vi "G.vi"(9 "5":string[](array[string]), 10 "4":string, 11 "A":string) -> (3 "G":string)   [LabVIEW 2017]
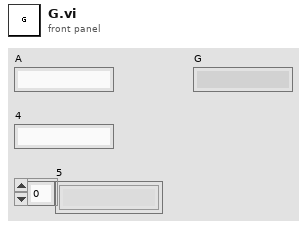
[diagram p1: front panel]
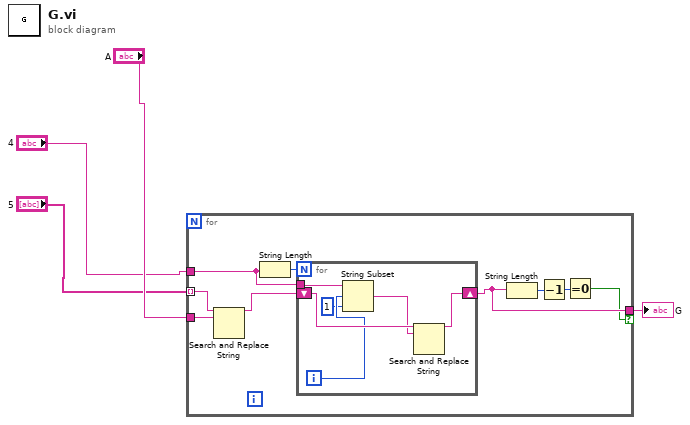
[diagram p0: block diagram]
diagram:
  n1 = for {
    tunnel: "5" -> [w7] mode=indexing
    tunnel: "4" -> [w12]
    tunnel: [w9] -> w3 if=w8
    tunnel: "A" -> [w5]
    n2 = Search and Replace String(input string=w7, search string=w5) -> (result string=w6:string)  [unwired: 6 in, 3 out]
    n3 = String Length(string=w12) -> (length=w13:i32)
    n4 = for {
      N: w13 -> [_]
      tunnel: w12 -> [w18]
      shift-right: [w14] -> w9
      shift-left: w6 -> [w19]
      i -> [w17]
      n5 = String Subset(string=w18, offset (0)=w17, length (rest)=1 ("length (rest)")) -> (substring=w15:string)
      n6 = Search and Replace String(input string=w19, search string=w15) -> (result string=w14:string)  [unwired: 6 in, 3 out]
    }
    n7 = String Length(string=w9) -> (length=w11:i32)
    n8 = Decrement(x=w11) -> (x-1=w10:i32)
    n9 = Equal To 0?(x=w10) -> (x = 0?=w8:bool)
  }
  "G" <- w3
